vi "Configure Channel Trigger Display.vi"(6 "Enable External Trigger Display (F: Disable)":bool, 8 "error in (no error)":errorcluster, 9 "Display Label (\"\")":string, 10 "Vertical Position (0)":dbl, 11 "VISA resource name":refnum<visa-resource-name>) -> (0 "error out":errorcluster, 3 "VISA resource name out":refnum<visa-resource-name>)   [LabVIEW 2016, in "Agilent 2000 3000 X-Series.lvlib"]
doc: "Specifies the external trigger display settings.\n\nNote: This VI is only applicable for 1000 X-Series."
uses:
  Agilent 2000 3000 X-Series.lvlib
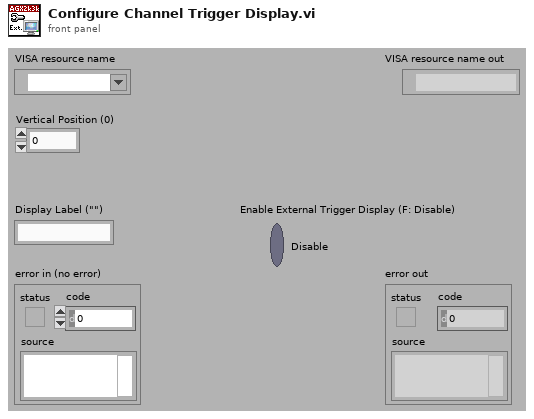
[diagram p1: front panel]
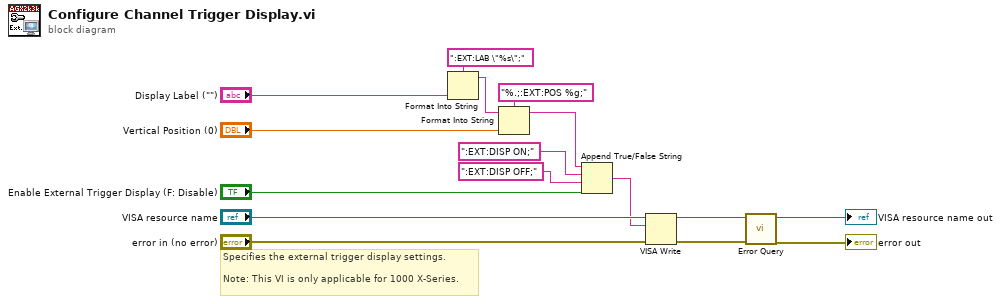
[diagram p0: block diagram]
diagram:
  # "Specifies the external trigger display settings.\n\nNote: This VI is only applicable for 1000 X-Series."
  n1 = Format Into String(format string=":EXT:LAB \"%s\";", "Display Label (\"\")") -> (resulting string=w14:string)  [unwired: 2 in, 1 out]
  n2 = Format Into String(format string="%.;:EXT:POS %g;", initial string=w14, "Vertical Position (0)") -> (resulting string=w2:string)  [unwired: 1 in, 1 out]
  n3 = Append True/False String(1:"Enable External Trigger Display (F: Disable)", 2:":EXT:DISP OFF;", 3:":EXT:DISP ON;", 4:w2) -> (0:w1:string)
  n4 = VISA Write(VISA resource name="VISA resource name", write buffer=w1, error in (no error)="error in (no error)") -> (VISA resource name out=w9:refnum<visa-resource-name>, error out=w8:errorcluster)  [unwired: 1 out]
  n5 = call "Error Query.vi"("error in (no error)"=w8, "VISA resource name"=w9) -> ("error out"=→"error out":errorcluster, "VISA resource name out"=→"VISA resource name out":refnum<visa-resource-name>)  [unwired: 6 in, 2 out]
